vi "RS232.vi"() -> ()   [LabVIEW 2012]
uses:
  <vilib>/Instr/_visa.llb/VISA Configure Serial Port (Instr).vi
  Globalna_Variabla.vi
panel:
  in  "Tab Control":enum32{"Setings", "Recived Data"}(tab)=enum."Recived Data"
  out "Read Buffer":string
  in  "VISA resource name":refnum<visa-resource-name>="COM18"
  in  "Baud Rate (9600)":u32=9600
  in  "Reciving Byte Count (9)":u32=9
  in  "length":i32=100
  in  "index":i32
  out "Buffer Index":i8
  out "Iteration":i32
  out "Recived bytes (5)":string[](array[string])
  out "String Output (4)":string[](array[string])
  in  "Split Index (5)":i32=5
  out "index of NaN":i32
  out "size(s)":i32
  in  "Sekvenca":dbl[](array[numeric])
  in  "Treshold":dbl=0.8
  out "Double Output (4)":dbl[](array[numeric])
  in  "stop":bool
  # "Brisanje Sekvence"
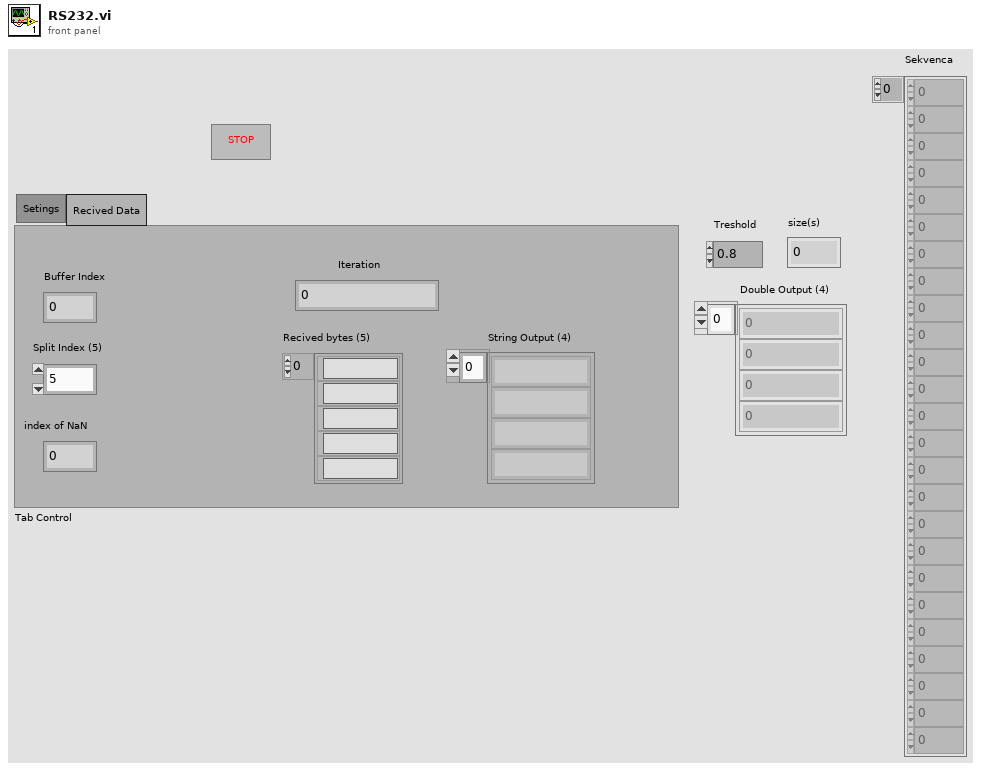
[diagram p1: front panel]
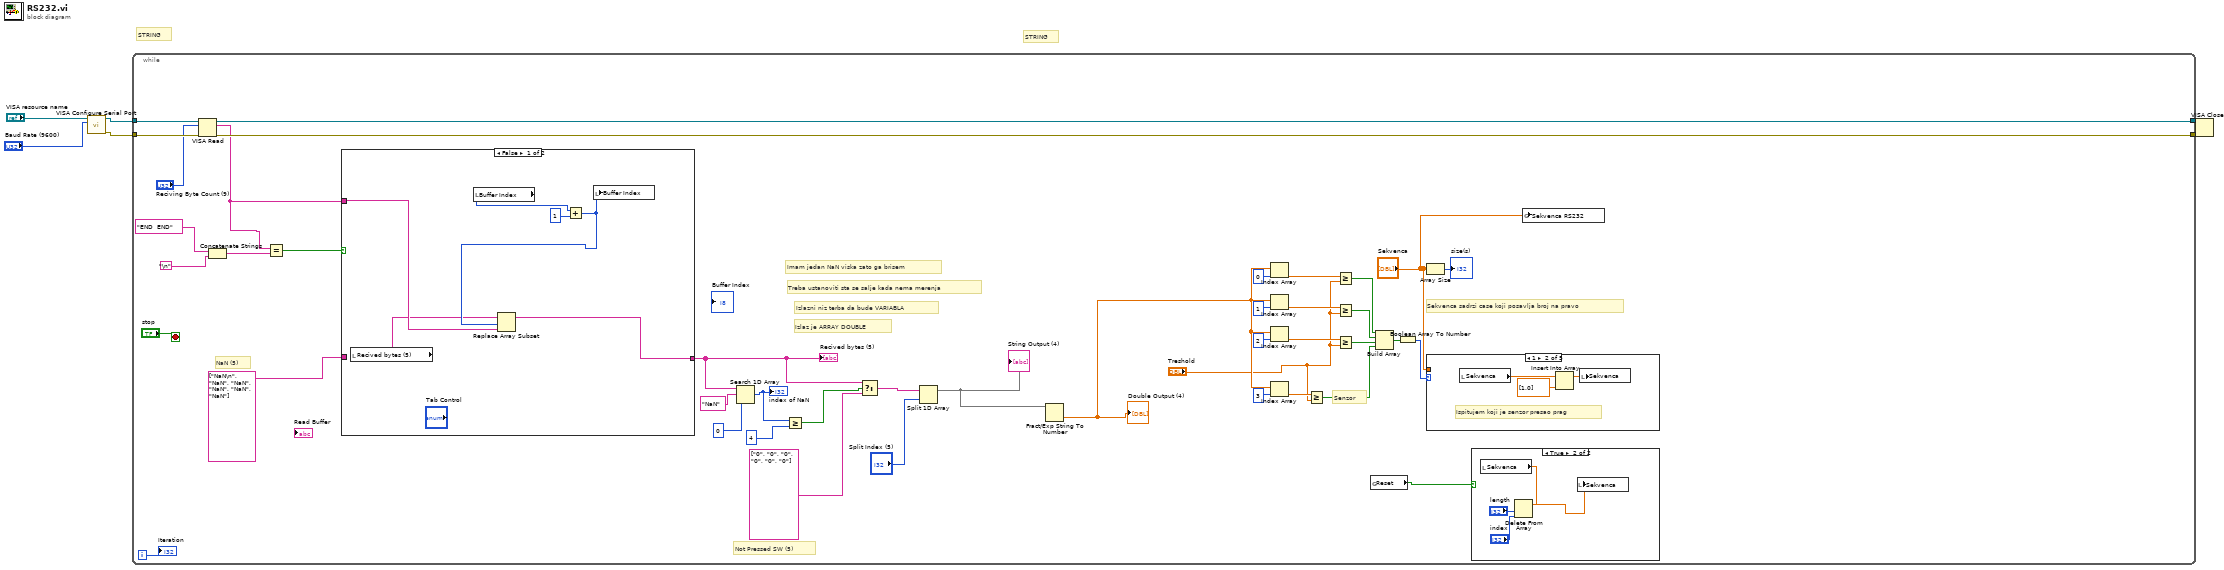
[diagram p0: block diagram]
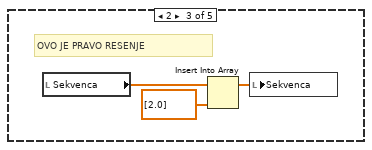
[diagram p4: hidden frame]
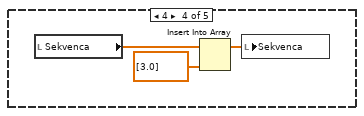
[diagram p5: hidden frame]
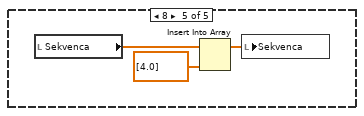
[diagram p6: hidden frame]
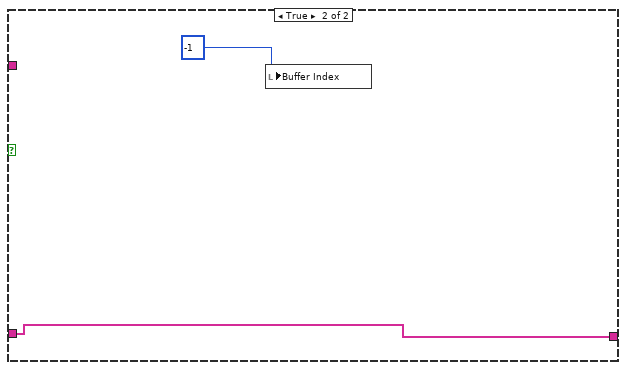
[diagram p7: hidden frame]
diagram:
  # "STRING"
  # "STRING"
  n1 = call-poly "VISA Configure Serial Port"("VISA resource name"="VISA resource name", "baud rate (9600)"="Baud Rate (9600)") -> ("VISA resource name out"=w5:refnum<visa-resource-name>, "error out"=w3:errorcluster)  [unwired: 12 in]
  n2 = while {
    tunnel: w5 -> [w47]
    tunnel: [w46] -> w4
    tunnel: w3 -> [w45]
    tunnel: [w44] -> w2
    i -> [w27]
    stop <- "stop" stop-if-true
    # "Senzor"
    # "Sekvenca sadrzi case koji posavlja broj na pravo"
    # "Izlaz je ARRAY DOUBLE"
    # "Izlazni niz terba da bude VARIABLA"
    # "NaN (5)"
    # "Not Pressed SW (5)"
    # "Treba ustanoviti sta se salje kada nema merenja"
    # "Imam jedan NaN viska zato ga brisem"
    n3 = VISA Read(VISA resource name=w47, byte count="Reciving Byte Count (9)", error in (no error)=w45) -> (VISA resource name out=w46:refnum<visa-resource-name>, read buffer=w39:string, error out=w44:errorcluster)  [unwired: 1 out]
    n4 = Concatenate Strings("END  END" ("y"), "\n") -> (w42:string)
    n5 = Equal?(x=w39, y=w42) -> (x = y?=w32:bool)
    n6 = case shown="False" w32 {
      tunnel: w39 -> [w66 _]
      tunnel: [w70 w71] -> w35
      tunnel: string[] ["NaN\n", "NaN", "NaN", "NaN", "NaN", "NaN"] -> [_ w71]
      frame False {
        n7 = local read "Recived bytes (5)"() -> (w65:string[])
        n8 = local read "Buffer Index"() -> (w68:i8)
        n9 = Add(x=w68, y=i8 1) -> (x+y=w67:i8)
        n10 = Replace Array Subset(array=w65, new element=w66, index=w67) -> (w70:string[])
        n11 = local write "Buffer Index"(w67) -> ()
      }
      frame True {
        n12 = local write "Buffer Index"(i8 -1 ("Numeric")) -> ()
      }
    }
    "Recived bytes (5)" <- w35
    n13 = Search 1D Array(1D array=w35, element="NaN", start index (0)=0) -> (index of element=w36:i32)
    "index of NaN" <- w36
    n14 = Greater Or Equal?(x=w36, y=4) -> (x >= y?=w34:bool)
    n15 = Select(t=w35, s=w34, f=string[] ["0", "0", "0", "0", "0", "0"]) -> (s? t:f=w31:string[])
    n16 = Split 1D Array(array=w31, index="Split Index (5)") -> (first subarray=w26:string[])  [unwired: 1 out]
    "String Output (4)" <- w26
    n17 = Fract/Exp String To Number(string=w26) -> (number=w10:dbl[])  [unwired: 3 in, 1 out]
    "Double Output (4)" <- w10
    n18 = Index Array(array=w10, index=0) -> (element=w14:dbl)
    n19 = Index Array(array=w10, index=1) -> (element=w13:dbl)
    n20 = Index Array(array=w10, index=2) -> (element=w12:dbl)
    n21 = Index Array(array=w10, index=3) -> (element=w11:dbl)
    n22 = Greater Or Equal?(x=w11, y="Treshold") -> (x >= y?=w18:bool)
    n23 = Greater Or Equal?(x=w14, y="Treshold") -> (x >= y?=w21:bool)
    n24 = Greater Or Equal?(x=w13, y="Treshold") -> (x >= y?=w20:bool)
    n25 = Greater Or Equal?(x=w12, y="Treshold") -> (x >= y?=w19:bool)
    n26 = global read "Globalna_Variabla.vi" "Reset"() -> (w7:bool)
    n27 = Build Array(w21, w20, w19, w18) -> (w17:bool[])
    n28 = Boolean Array To Number(Boolean array=w17) -> (number=w16:u32)
    n29 = Array Size(array="Sekvenca") -> (size(s)=→"size(s)":i32)
    n30 = case shown="1" w16 {
      tunnel: "Sekvenca" -> [_ _ _ _ _]
      frame 0, Default {
      }
      frame 1 {
        # "Ispitujem koji je senzor presao prag"
        n31 = local read "Sekvenca"() -> (w53:dbl[])
        n32 = Insert Into Array(array=w53, new element=dbl[] [1.0]) -> (w55:dbl[])  [unwired: 1 in]
        n33 = local write "Sekvenca"(w55) -> ()
      }
      frame 2 {
        # "OVO JE PRAVO RESENJE"
        n34 = local read "Sekvenca"() -> (w56:dbl[])
        n35 = Insert Into Array(array=w56, new element=dbl[] [2.0]) -> (w58:dbl[])  [unwired: 1 in]
        n36 = local write "Sekvenca"(w58) -> ()
      }
      frame 4 {
        n37 = local read "Sekvenca"() -> (w59:dbl[])
        n38 = Insert Into Array(array=w59, new element=dbl[] [3.0]) -> (w61:dbl[])  [unwired: 1 in]
        n39 = local write "Sekvenca"(w61) -> ()
      }
      frame 8 {
        n40 = local read "Sekvenca"() -> (w62:dbl[])
        n41 = Insert Into Array(array=w62, new element=dbl[] [4.0]) -> (w64:dbl[])  [unwired: 1 in]
        n42 = local write "Sekvenca"(w64) -> ()
      }
    }
    n43 = case shown="True" w7 {
      frame False {
      }
      frame True {
        n44 = local read "Sekvenca"() -> (w51:dbl[])
        n45 = Delete From Array(array=w51, length="length", index="index") -> (array with subset deleted=w52:dbl[])  [unwired: 1 out]
        n46 = local write "Sekvenca"(w52) -> ()
      }
    }
    n47 = global write "Globalna_Variabla.vi" "Sekvenca RS232"("Sekvenca") -> ()
    "Iteration" <- w27
  }
  n48 = VISA Close(VISA resource name=w4, error in (no error)=w2) -> ()  [unwired: 1 out]
